vi "time_as_file_name.vi"() -> (2 "Path":path, 3 "Filename":string)   [LabVIEW 2020]
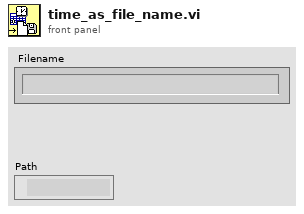
[diagram p1: front panel]
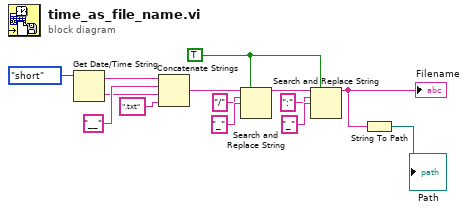
[diagram p0: block diagram]
diagram:
  w10 = TRUE ("replace all? (F)")
  n1 = Get Date/Time String(date format (0)=enum16{"short", "long", "abbreviated"}."short") -> (date string=w2:string, time string=w11:string)  [unwired: 2 in]
  n2 = Concatenate Strings(w2, "__" ("string"), w11, ".txt") -> (w4:string)
  n3 = Search and Replace String(replace all?=w10, input string=w4, search string="/", replace string="_" ("replace string (\"\")")) -> (result string=w7:string)  [unwired: 4 in, 3 out]
  n4 = Search and Replace String(replace all?=w10, input string=w7, search string=":", replace string="_" ("replace string (\"\")")) -> (result string=w14:string)  [unwired: 4 in, 3 out]
  "Filename" <- w14
  n5 = String To Path(string=w14) -> (path=→"Path":path)
